vi "transform_lut.vi"(9 "Demodulated signals":waveform(sgl)[][](array[waveform])) -> (0 "Sum amplitudes":sgl[][](array[numeric]), 1 "Match error":waveform(sgl)[](array[waveform]), 3 "XYZ out":T1(array[cluster]), 4 "Axis positions":sgl[][](array[numeric]))   [LabVIEW 2012]
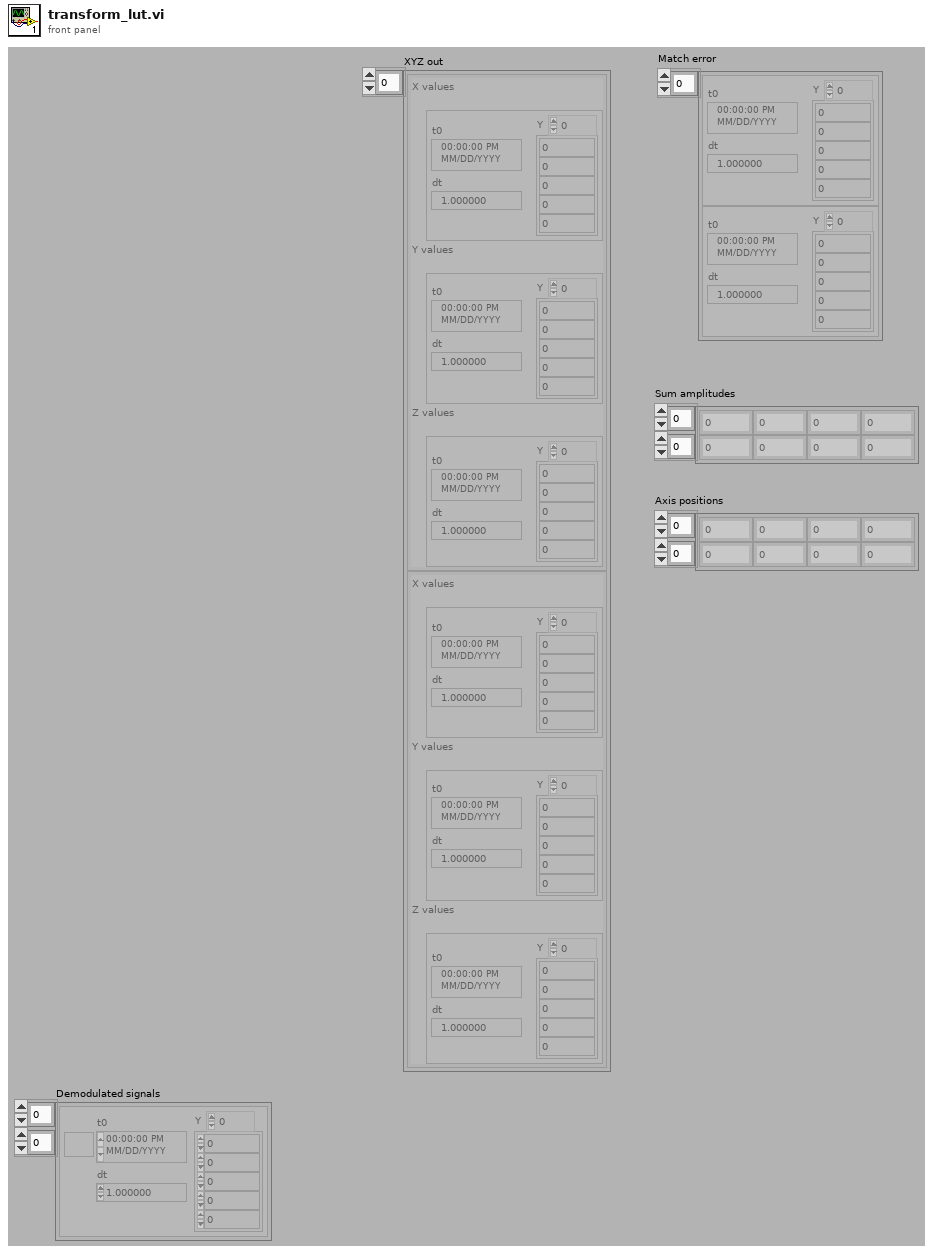
[diagram p1: front panel]
types:
  T1 = cluster{"X values":waveform(sgl), "Y values":waveform(sgl), "Z values":waveform(sgl)}[]
  T2 = cluster{"[0]":waveform(sgl), "[1]":waveform(sgl), "[2]":waveform(sgl)}
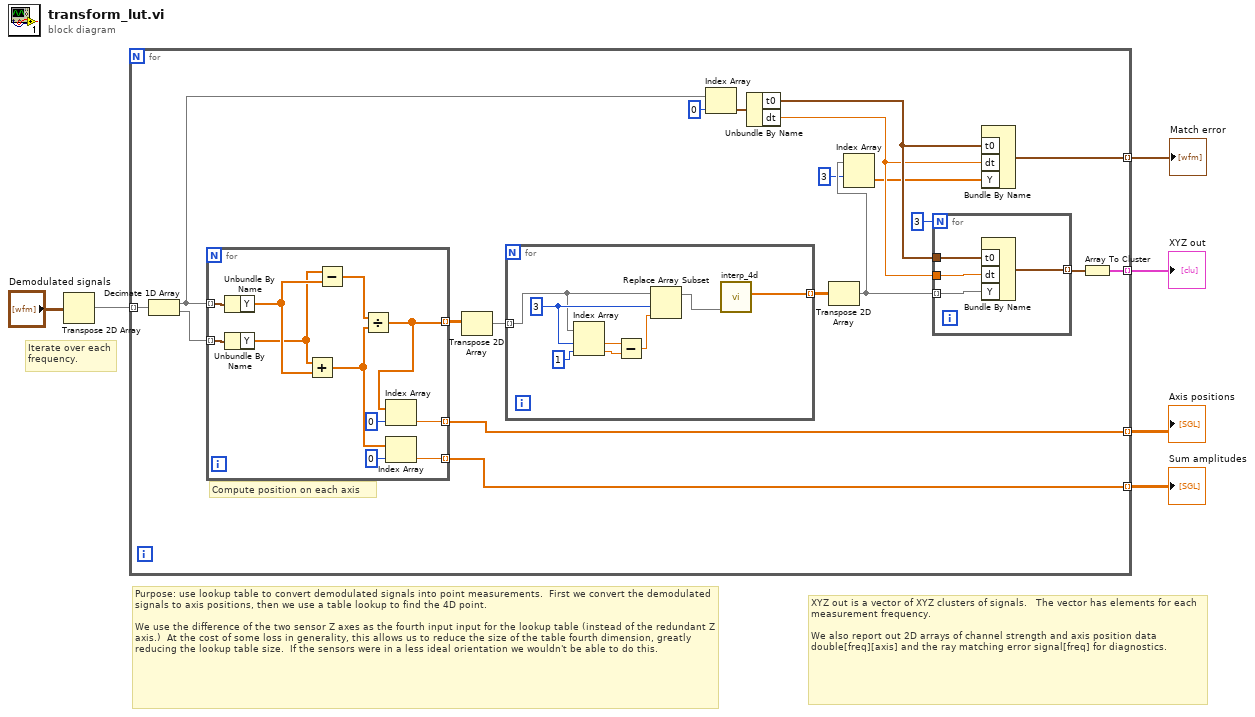
[diagram p0: block diagram]
diagram:
  # "Purpose: use lookup table to convert demodulated signals into point measurements.  First we convert the demodulated signals to axis positions, then we use a table lookup to find the 4D point.\n\nWe use the difference of the two sensor Z axes as the fourth input input for the lookup table (instead of the redundant Z axis.)  At the cost of some loss in generality, this allows us to reduce the size of the table fourth dimension, greatly reducing the lookup table size.  If the sensors were in a less ideal orientation we wouldn't be able to do this."
  # "XYZ out is a vector of XYZ clusters of signals.   The vector has elements for each measurement frequency. \n\nWe also report out 2D arrays of channel strength and axis position data double[freq][axis] and the ray matching error signal[freq] for diagnostics."
  # "Iterate over each\nfrequency."
  n1 = Transpose 2D Array(2D array="Demodulated signals") -> (transposed array=w5:waveform(sgl)[][])
  n2 = for {
    tunnel: w5 -> [w25] mode=indexing
    tunnel: [w23] -> w4 mode=indexing
    tunnel: [w19] -> w3 mode=indexing
    tunnel: [w14] -> w2 mode=indexing
    tunnel: [w11] -> w1 mode=indexing
    # "Compute position on each axis"
    n3 = Decimate 1D Array(w25) -> (w22:waveform(sgl)[], w24:waveform(sgl)[])
    n4 = for {
      tunnel: [w39] -> w18 mode=indexing
      tunnel: w22 -> [w47] mode=indexing
      tunnel: w24 -> [w46] mode=indexing
      tunnel: [w43] -> w23 mode=indexing
      tunnel: [w38] -> w19 mode=indexing
      n5 = Unbundle By Name(w47) -> ("Y"=w42:sgl[])
      n6 = Unbundle By Name(w46) -> ("Y"=w41:sgl[])
      n7 = Add(x=w41, y=w42) -> (x+y=w45:sgl[])
      n8 = Subtract(x=w41, y=w42) -> (x-y=w48:sgl[])
      n9 = Divide(x=w48, y=w45) -> (x/y=w39:sgl[])
      n10 = Index Array(array=w39, index=0) -> (element=w38:sgl)
      n11 = Index Array(array=w45, index=0) -> (element=w43:sgl)
    }
    n12 = Transpose 2D Array(2D array=w18) -> (transposed array=w17:sgl[][])
    n13 = for {
      tunnel: w17 -> [w31] mode=indexing
      tunnel: [w37] -> w16 mode=indexing
      w32 = 3 ("index (row)")
      n14 = Index Array(array=w31, index #1=w32, index #2=1 ("index (row)")) -> (element #1=w34:sgl, element #2=w35:sgl)
      n15 = Subtract(x=w34, y=w35) -> (x-y=w36:sgl)
      n16 = Replace Array Subset(array=w31, new element=w36, index=w32) -> (w30:sgl[])
      n17 = call "interp_4d.vi"("Input x"=w30) -> ("Output f(x)"=w37:sgl[])  [unwired: 2 in, 8 out]
    }
    n18 = Index Array(array=w22, index=0) -> (element=w20:waveform(sgl))
    n19 = Unbundle By Name(w20) -> ("t0"=w13:timestamp, "dt"=w12:dbl)
    n20 = Transpose 2D Array(2D array=w16) -> (transposed array=w9:sgl[][])
    n21 = Index Array(array=w9, index (row)=3) -> (element=w7:sgl[])  [unwired: 1 in]
    n22 = for {
      N: 3 -> [_]
      tunnel: w9 -> [w29] mode=indexing
      tunnel: w12 -> [w28]
      tunnel: w13 -> [w27]
      tunnel: [w26] -> w15 mode=indexing
      n23 = Bundle By Name("t0"=w27, "dt"=w28, "Y"=w29) -> (w26:waveform(sgl))  [unwired: 1 out]
    }
    n24 = Bundle By Name("t0"=w13, "dt"=w12, "Y"=w7) -> (w11:waveform(sgl))  [unwired: 1 out]
    n25 = Array To Cluster(array=w15) -> (cluster=w14:T2)
  }
  "XYZ out" <- w2
  "Sum amplitudes" <- w4
  "Match error" <- w1
  "Axis positions" <- w3
